vi "Process.vi"(8 "error in (no error)":errorcluster, 11 "RandomNumberLogger in":refnum<class "RandomNumberLogger.lvclass">) -> (0 "error out":errorcluster, 3 "RandomNumberLogger out":refnum<class "RandomNumberLogger.lvclass">)   [LabVIEW 2020, in "RandomNumberLogger.lvlib" / "RandomNumberLogger.lvclass"]
doc: "<b>Process</b>\nThis method is called based on the timing set in the <b>Initialize</b> or <b>Configure Session</b> methods, and is where the vast majority of the work done by your plugin will happen. Here, your plugin can read the data that was sent to the plugin (if any), perform some action(s), and optionally send data to the PEF Engine for other plugins to receive.\n\nThe Process state gets called repeatedly by the engine. You do not need to implement a while loop to continuously run in the Process state. Your process state must not call any code with an infinite timeout. \nInstead, use a defined timeout and handle/ignore the timeout error accordingly. This ensures that the system does not hang or get stuck.\n\nThere may be many instances of the same plugin running on the system. Because the state VIs in plugins run with Shared Clone reentrancy, there is no guarantee that any data stored in diagram or front panel structures (such as feedback nodes, shift registers, front panel objects, etc) are from the same instance of the plugin. Any data that needs to persist between calls to the Process VI must be persisted in the class private data of the plugin."
uses:
  RandomNumberLogger.lvclass
  C:/Program Files/National Instruments/LabVIEW 2020/vi.lib/FlexLogger/SDK/PluginSDK.lvlibp/PEFClasses/SDK/Processing Element/Processing Element.lvclass
  RandomNumberLogger.lvclass/RandomNumberLogger.ctl
  Read Configuration.vi
  <vilib>/FlexLogger/SDK/PluginSDK.lvlibp/PEFClasses/SDK/Processing Element/Read Alias.vi
  <vilib>/ADAS Record/pefCommon/Tracing/SendGenericEvent.vi
  <vilib>/FlexLogger/SDK/PluginSDK.lvlibp/PEFClasses/SDK/Processing Element/Read System Interface.vi
  <vilib>/ADAS Record/CustomDataTypes/Double/Read.vi
  <vilib>/FlexLogger/SDK/PluginSDK.lvlibp/PEFClasses/SDK/System Interface/System Interface.lvclass
  <vilib>/ADAS Record/Utilities/ADAS Utilities.lvlib
  <vilib>/ADAS Record/CustomDataTypes/Double/Double.lvlib
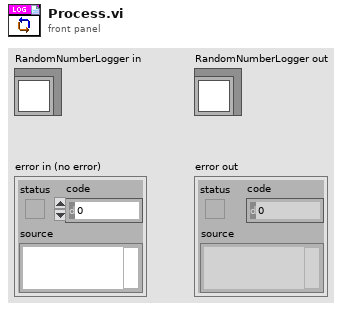
[diagram p1: front panel]
types:
  T1 = typedef "RandomNumberLogger.lvlib/RandomNumberLogger.lvclass/Configuration.ctl" = cluster{"Base File Name":string, "File Directory":path, "File Split":enum16{"None", "Time", "Size"}, "Split Time/Size (sec/MB)":dbl}
  T2 = typedef "Double.lvlib/Process Data.ctl" = cluster{"Time Stamp":timestamp, "Double (DBL)":dbl}
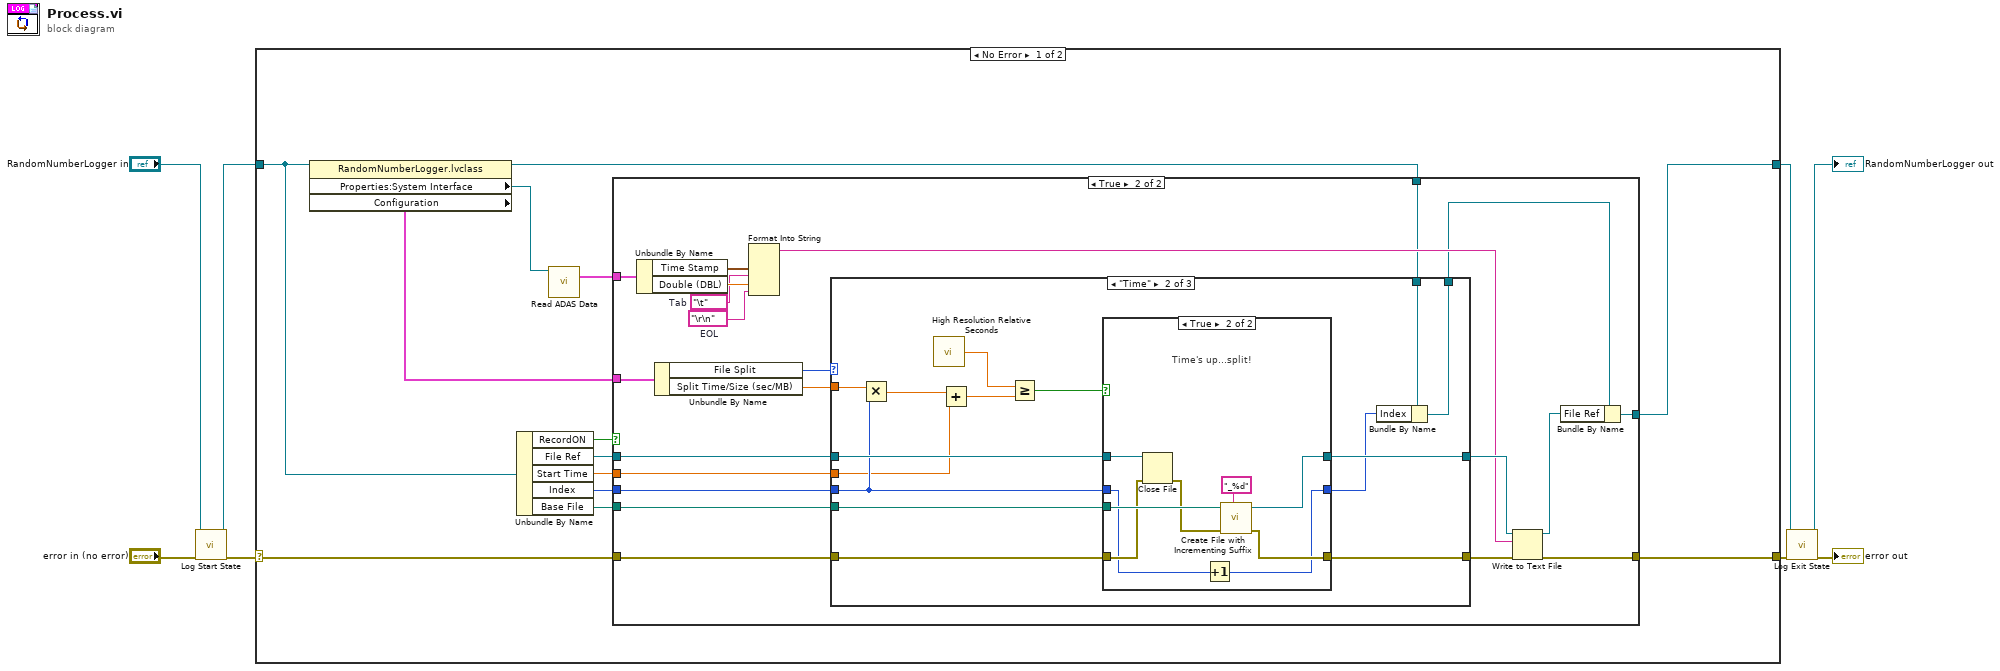
[diagram p0: block diagram]
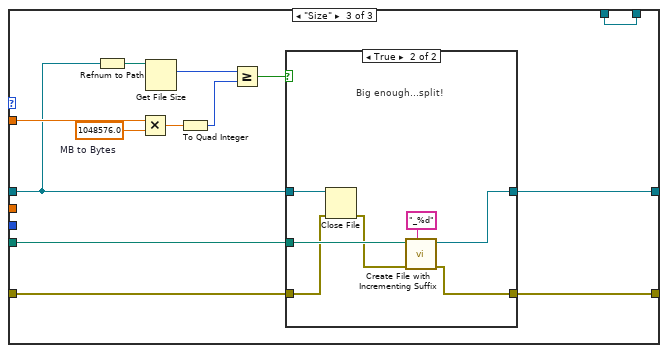
[diagram p5: hidden frame]
diagram:
  n1 = call <vilib>:"Log Start State.vi"("error in (no error)"="error in (no error)", "PluginSDK.lvlibp:Processing Element.lvclass"="RandomNumberLogger in") -> ("error out"=w7:errorcluster, "PluginSDK.lvlibp:Processing Element.lvclass"=w5:refnum<class "RandomNumberLogger.lvclass">)  [unwired: 8 in]
  n2 = case shown="No Error" w7 {
    selector: w7 -> [w19 w97]
    tunnel: [w11 w98] -> w2
    tunnel: w5 -> [w17 w98]
    tunnel: [w10 w97] -> w4
    frame No Error {
      n3 = property on="Property Node" class="RandomNumberLogger.lvclass"(reference=w17) -> (reference out=w9:refnum<class "RandomNumberLogger.lvclass">, "Properties:System Interface"=w21:refnum<class "System Interface.lvclass">, "Configuration"=w18:T1)  [unwired: 1 in, 1 out]
      n4 = Unbundle By Name(w17) -> ("RecordON"=w16:bool, "File Ref"=w15:refnum<file>, "Start Time"=w14:dbl, "Index"=w13:u64, "Base File"=w12:path)
      n5 = call-poly <vilib>:"Read ADAS Data.vi"("System Interface in"=w21) -> ("Process Data"=w20:T2)  [unwired: 12 in, 2 out]
      n6 = case shown="True" w16 {
        tunnel: w20 -> [_ w44]
        tunnel: w19 -> [w23 w38]
        tunnel: w18 -> [_ w39]
        tunnel: w15 -> [_ w31]
        tunnel: w14 -> [_ w27]
        tunnel: w13 -> [_ w28]
        tunnel: w12 -> [_ w29]
        tunnel: [w22 w35] -> w11
        tunnel: [w23 w33] -> w10
        tunnel: w9 -> [w22 w25]
        frame False {
        }
        frame True {
          w40 = "\r\n"  # EOL
          w41 = "\t"  # Tab
          n7 = Unbundle By Name(w44) -> ("Time Stamp"=w43:timestamp, "Double (DBL)"=w42:dbl)
          n8 = Unbundle By Name(w39) -> ("File Split"=w37:enum16{"None", "Time", "Size"}, "Split Time/Size (sec/MB)"=w30:dbl)
          n9 = Format Into String(w43, w41, w42, w40) -> (resulting string=w26:string)  [unwired: 3 in, 1 out]
          n10 = case shown="\"Time\"" w37 {
            tunnel: [w46 w60 w76] -> w34
            tunnel: w38 -> [w46 w61 w77]
            tunnel: [w47 w62 w79] -> w32
            tunnel: w31 -> [w47 w59 w78]
            tunnel: w30 -> [_ w53 w86]
            tunnel: w29 -> [_ w58 w81]
            tunnel: w28 -> [_ w52 _]
            tunnel: w27 -> [_ w51 _]
            tunnel: w25 -> [w45 w57 w75]
            tunnel: [w45 w56 w75] -> w24
            frame "None", Default {
            }
            frame "Time" {
              n11 = Multiply(x=w53, y=w52) -> (x*y=w50:dbl)
              n12 = call <vilib>:"High Resolution Relative Seconds.vi"() -> ("relative seconds"=w54:dbl)
              n13 = Add(x=w50, y=w51) -> (x+y=w49:dbl)
              n14 = Greater Or Equal?(x=w54, y=w49) -> (x >= y?=w48:bool)
              n15 = case shown="True" w48 {
                tunnel: w58 -> [_ w74]
                tunnel: [w65 w72] -> w62
                tunnel: w59 -> [w65 w70]
                tunnel: w61 -> [w64 w69]
                tunnel: [w64 w71] -> w60
                tunnel: w52 -> [w63 w67]
                tunnel: [w63 w66] -> w55
                frame False {
                }
                frame True {
                  # "Time's up...split!"
                  n16 = Close File(refnum=w70, error in=w69) -> (error out=w68:errorcluster)  [unwired: 1 out]
                  n17 = Increment(x=w67) -> (x+1=w66:u64)
                  n18 = call <vilib>:"Create File with Incrementing Suffix.vi"("format string (\" (%d)\")"="_%d" ("format string (\" (%d)\")"), "error in (no error)"=w68, "file path"=w74) -> ("error out"=w71:errorcluster, "refnum out"=w72:refnum<file>)  [unwired: 6 in, 1 out]
                }
              }
              n19 = Bundle By Name(cluster=w57, "Index"=w55) -> (w56:refnum<class "RandomNumberLogger.lvclass">)
            }
            frame "Size" {
              w85 = 1048576.0  # MB to Bytes
              n20 = Refnum to Path(1:w78) -> (0:w87:path)
              n21 = Multiply(x=w86, y=w85) -> (x*y=w83:dbl)
              n22 = Get File Size(file=w87) -> (size (in bytes)=w84:i64)  [unwired: 1 in, 2 out]
              n23 = To Quad Integer(1:w83) -> (0:w82:i64)
              n24 = Greater Or Equal?(x=w84, y=w82) -> (x >= y?=w80:bool)
              n25 = case shown="True" w80 {
                tunnel: w81 -> [_ w96]
                tunnel: [w89 w94] -> w79
                tunnel: w78 -> [w89 w92]
                tunnel: w77 -> [w88 w91]
                tunnel: [w88 w93] -> w76
                frame False {
                }
                frame True {
                  # "Big enough...split!"
                  n26 = Close File(refnum=w92, error in=w91) -> (error out=w90:errorcluster)  [unwired: 1 out]
                  n27 = call <vilib>:"Create File with Incrementing Suffix.vi"("format string (\" (%d)\")"="_%d" ("format string (\" (%d)\")"), "error in (no error)"=w90, "file path"=w96) -> ("error out"=w93:errorcluster, "refnum out"=w94:refnum<file>)  [unwired: 6 in, 1 out]
                }
              }
            }
          }
          n28 = Write to Text File(file (use dialog)=w32, text=w26, error in=w34) -> (refnum out=w36:refnum<file>, error out=w33:errorcluster)  [unwired: 1 in, 1 out]
          n29 = Bundle By Name(cluster=w24, "File Ref"=w36) -> (w35:refnum<class "RandomNumberLogger.lvclass">)
        }
      }
    }
    frame Error {
    }
  }
  n30 = call <vilib>:"Log Exit State.vi"("error in (no error)"=w4, "PluginSDK.lvlibp:Processing Element.lvclass"=w2) -> ("error out"=→"error out":errorcluster, "PluginSDK.lvlibp:Processing Element.lvclass"=→"RandomNumberLogger out":refnum<class "RandomNumberLogger.lvclass">)  [unwired: 8 in]
